vi "Project - Options.vi"(7 "Msg Chain":string, 8 "error in (no error)":errorcluster {"code" format="Error %.0f"}, 10 "Project Doc":refnum<class "Project Documentation.lvclass">, 11 "VIDoc Printer - Confluence In":refnum<class "VIDoc Printer - Confluence.lvclass">) -> (0 "error out":errorcluster {"code" format="Error %.0f"}, 3 "VIDoc Printer - Confluence Out":refnum<class "VIDoc Printer - Confluence.lvclass">)   [LabVIEW 2023, in "VIDoc Printer - Confluence.lvlib" / "VIDoc Printer - Confluence.lvclass"]
uses:
  VIDoc Printer - Confluence.lvclass
  Parsing/Project Documentation/Project Documentation.lvclass
  Confluence Formatting/Types/Format Combo Box.ctl
  Parsing/Project Documentation/Project Documentation.lvclass/Project Documentation.ctl
  Parsing/Project Documentation/Get SCC.vi
  VIDoc Printer - Confluence.lvclass/VIDoc Printer - Confluence.ctl
  Confluence Formatting/Confluence Formatting.lvlib
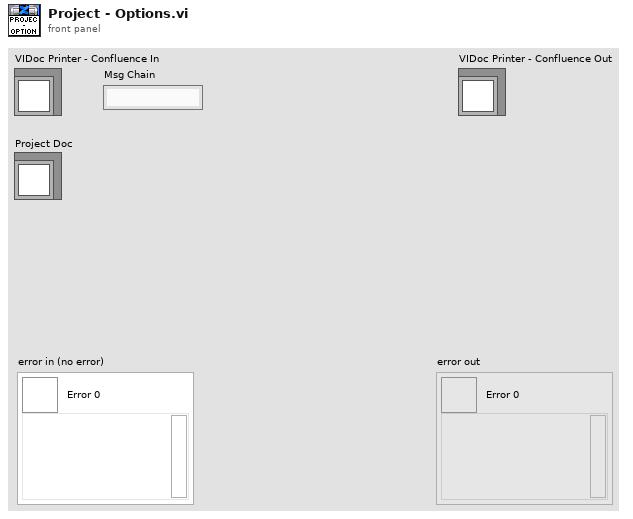
[diagram p1: front panel]
types:
  T1 = typedef "Confluence Formatting.lvlib/Format Combo Box.ctl" = string
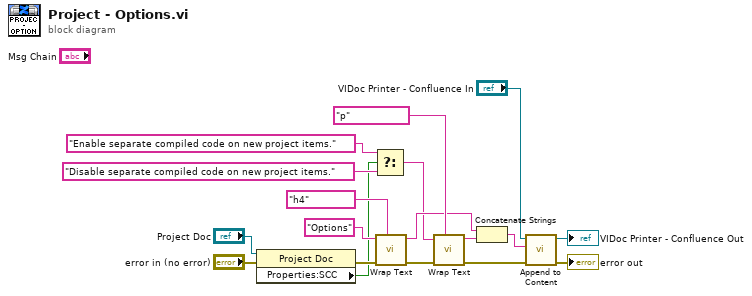
[diagram p0: block diagram]
diagram:
  n1 = property class="Project Doc"(reference="Project Doc", error in="error in (no error)") -> (error out=w15:errorcluster, "Properties:SCC"=w2:bool)  [unwired: 1 out]
  n2 = Select(t="Enable separate compiled code on new project items.", s=w2, f="Disable separate compiled code on new project items.") -> (s? t:f=w1:string)
  n3 = call "Wrap Text.vi"("Formatting"=T1 "h4", "Error in"=w15, "String"="Options") -> ("Error out"=w12:errorcluster, "Wrapped String"=w14:string)  [unwired: 7 in]
  n4 = call "Wrap Text.vi"("Formatting"=T1 "p", "Error in"=w12, "String"=w1) -> ("Error out"=w11:errorcluster, "Wrapped String"=w13:string)  [unwired: 7 in]
  n5 = Concatenate Strings(w14, w13) -> (w10:string)
  n6 = call "Append to Content.vi"("error in (no error)"=w11, "Content"=w10, "VIDoc Printer - Confluence In"="VIDoc Printer - Confluence In") -> ("error out"=→"error out":errorcluster, "VIDoc Printer - Confluence Out"=→"VIDoc Printer - Confluence Out":refnum<class "VIDoc Printer - Confluence.lvclass">)  [unwired: 7 in]
